vi "Column Timestamp.vi"(8 "error in (no error)":errorcluster, 11 "SQL Statement in":refnum<class "SQL Statement.lvclass">) -> (0 "error out":errorcluster, 2 "Time Stamp":timestamp, 3 "SQL Statement out":refnum<class "SQL Statement.lvclass">)   [LabVIEW 2011, in "SQLite.lvlib" / "SQL Statement.lvclass"]
doc: "Extracts a Timestamp. There is no SQLite3 datatype for Timestamps. This function attempts to convert from the following formats:\n\n1) A standard 128bit LabVIEW Timestamp in a 16-byte BLOB.\n\n2) A LabVIEW Timestamp converted to a DBL, stored in a FLOAT.\n\n3) A timestring stored as TEXT, in the general format \"YYYY-MM-DD HH:MM:SS.SSS\" \npartial seconds are optional. The space can be replaced with a \"T\". Times are assumed to be UTC, regardless of whether this is indicated by a \"Z\" at the end. Reference the ISO8601 standard."
uses:
  SQL Statement.lvclass
  SQL Statement.lvclass/SQL Statement.ctl
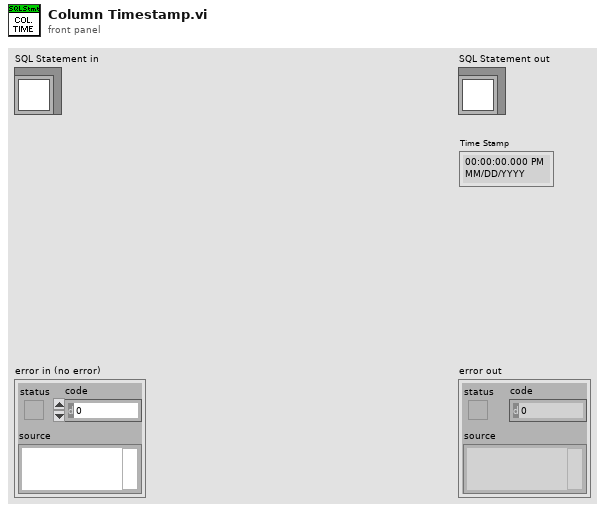
[diagram p1: front panel]
types:
  T1 = typedef "SQLite.lvlib/SQLITE Datatype.ctl" = enum32{"undefined type (0)", "SQLITE_INTEGER", "SQLITE_FLOAT", "SQLITE3_TEXT", "SQLITE_BLOB", "SQLITE_NULL", "undefined type"}
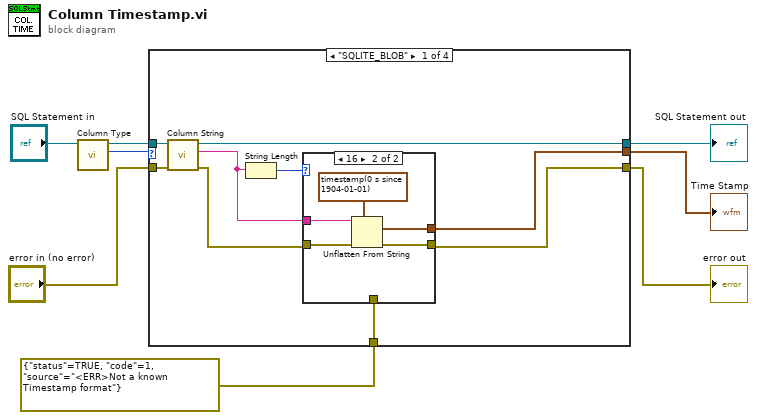
[diagram p0: block diagram]
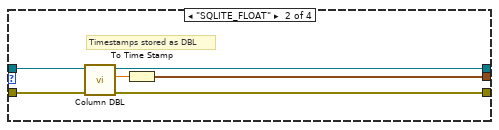
[diagram p3: hidden frame]
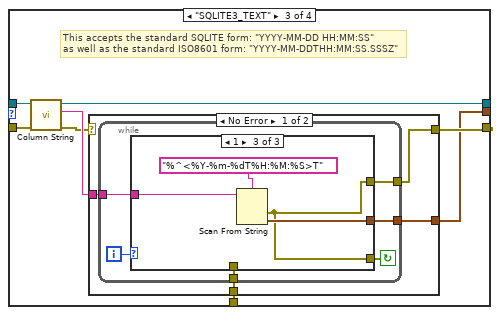
[diagram p4: hidden frame]
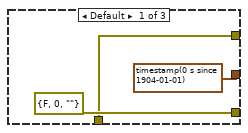
[diagram p5: hidden frame]
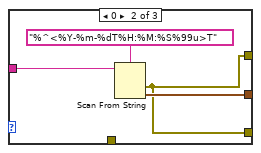
[diagram p6: hidden frame]
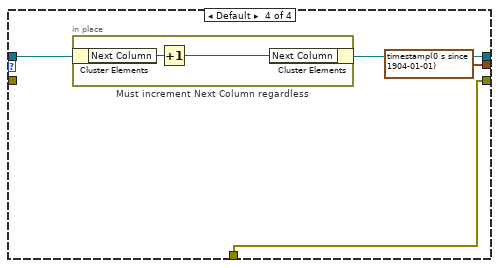
[diagram p8: hidden frame]
diagram:
  n1 = call "Column Type.vi"("SQL Statement in"="SQL Statement in") -> ("SQLite3 type"=w2:T1, "SQL Statement out"=w3:refnum<class "SQL Statement.lvclass">)  [unwired: 8 in, 1 out]
  n2 = case shown="\"SQLITE_BLOB\"" w2 {
    tunnel: [w17 w29 w37 w60] -> w8
    tunnel: "error in (no error)" -> [w16 w28 w36 _]
    tunnel: [w10 w27 w32 w63] -> w6
    tunnel: [w11 w26 w30 timestamp(0 s since 1904-01-01)] -> w5
    tunnel: w3 -> [w15 w24 w35 w61]
    tunnel: errorcluster {"status"=TRUE, "code"=1, "source"="<ERR>Not a known Timestamp format"} ("error out") -> [w9 _ w31 w63]
    frame "SQLITE_BLOB" {
      n3 = call "Column String.vi"("error in (no error)"=w16, "SQL Statement in"=w15) -> ("error out"=w12:errorcluster, "Text"=w13:string, "SQL Statement out"=w17:refnum<class "SQL Statement.lvclass">)  [unwired: 7 in]
      n4 = String Length(string=w13) -> (length=w14:i32)
      n5 = case shown="16" w14 {
        tunnel: w13 -> [_ w23]
        tunnel: w12 -> [_ w21]
        tunnel: [_ w20] -> w11
        tunnel: [w18 w19] -> w10
        tunnel: w9 -> [w18 _]
        frame Default {
        }
        frame 16 {
          n6 = Unflatten From String(type=timestamp(0 s since 1904-01-01), binary string=w23, error in (no error)=w21) -> (value=w20:timestamp, error out=w19:errorcluster)  [unwired: 2 in, 1 out]
        }
      }
    }
    frame "SQLITE_FLOAT" {
      # "Timestamps stored as DBL"
      n7 = call "Column DBL.vi"("error in (no error)"=w28, "SQL Statement in"=w24) -> ("error out"=w27:errorcluster, "DBL"=w25:dbl, "SQL Statement out"=w29:refnum<class "SQL Statement.lvclass">)  [unwired: 7 in]
      n8 = To Time Stamp(1:w25) -> (0:w26:timestamp)
    }
    frame "SQLITE3_TEXT" {
      # "This accepts the standard SQLITE form: \"YYYY-MM-DD HH:MM:SS\" \nas well as the standard ISO8601 form: \"YYYY-MM-DDTHH:MM:SS.SSSZ\""
      n9 = call "Column String.vi"("error in (no error)"=w36, "SQL Statement in"=w35) -> ("error out"=w33:errorcluster, "Text"=w34:string, "SQL Statement out"=w37:refnum<class "SQL Statement.lvclass">)  [unwired: 7 in]
      n10 = case shown="No Error" w33 {
        selector: w33 -> [_ w59]
        tunnel: w34 -> [w41 _]
        tunnel: [w40 w59] -> w32
        tunnel: w31 -> [w39 _]
        tunnel: [w38 _] -> w30
        frame No Error {
          n11 = while {
            tunnel: [w46] -> w38
            tunnel: [w44] -> w40
            tunnel: w41 -> [w43]
            tunnel: w39 -> [w42]
            i -> [w47]
            stop <- w45 continue-if-true
            n12 = case shown="1" w47 {
              tunnel: [timestamp(0 s since 1904-01-01) w53 w57] -> w46
              tunnel: [errorcluster {"status"=FALSE, "code"=0, "source"=""} ("error IO") w52 w56] -> w45
              tunnel: [w48 w52 w56] -> w44
              tunnel: w43 -> [_ w51 w55]
              tunnel: w42 -> [w48 _ _]
              frame Default {
              }
              frame 0 {
                n13 = Scan From String(format string="%^<%Y-%m-%dT%H:%M:%S%99u>T", input string=w51) -> (error out=w52:errorcluster, output 1=w53:timestamp)  [unwired: 3 in, 2 out]
              }
              frame 1 {
                n14 = Scan From String(format string="%^<%Y-%m-%dT%H:%M:%S>T", input string=w55) -> (error out=w56:errorcluster, output 1=w57:timestamp)  [unwired: 3 in, 2 out]
              }
            }
          }
        }
        frame Error {
        }
      }
    }
    frame Default {
      n15 = in-place "Must increment Next Column regardless" {
        n16 = in-place-cluster #1(w61) -> ("Next Column"=w65:i32)
        n17 = Increment(x=w65) -> (x+1=w64:i32)
        n18 = in-place-cluster #1("Next Column"=w64) -> (w60:refnum<class "SQL Statement.lvclass">)
      }
    }
  }
  "error out" <- w6
  "SQL Statement out" <- w8
  "Time Stamp" <- w5
